vi "reshape 1D stream into 2D channel array.vi"(10 "FIFIO channel count":i32, 11 "1D datastream in":dbl[](array[numeric])) -> (2 "dataPoints":i32, 3 "2D data array out":dbl[][](array[numeric]))   [LabVIEW 2018]
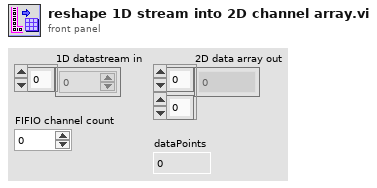
[diagram p1: front panel]
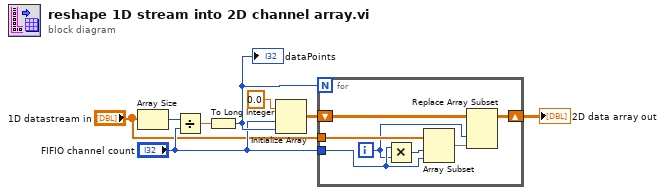
[diagram p0: block diagram]
diagram:
  n1 = Array Size(array="1D datastream in") -> (size(s)=w1:i32)
  n2 = Divide(x=w1, y="FIFIO channel count") -> (x/y=w2:dbl)
  n3 = To Long Integer(number=w2) -> (32bit integer=w8:i32)
  "dataPoints" <- w8
  n4 = Initialize Array(0.0 ("raw data"), "FIFIO channel count", w8) -> (w5:dbl[][])
  n5 = for {
    N: w8 -> [_]
    tunnel: "1D datastream in" -> [w15]
    shift-right: [w10] -> w6
    shift-left: w5 -> [w12]
    tunnel: "FIFIO channel count" -> [w13]
    i -> [w9]
    n6 = Multiply(x=w13, y=w9) -> (x*y=w14:i32)
    n7 = Array Subset(array=w15, index=w14, length=w13) -> (w11:dbl[])
    n8 = Replace Array Subset(array=w12, new element=w11, index (col)=w9) -> (w10:dbl[][])  [unwired: 1 in]
  }
  "2D data array out" <- w6
